vi "broadcast_ping.vi"() -> ()   [LabVIEW 2015]
uses:
  dxl_x86_c.lvlib/dxl_x86_c.lvlib
panel:
  in  "dynamixel_id_list":string[][](table)
  in  "device_name":string="COM8"
  out "protocol_version":dbl=2.0
  out "port_num":i32
  in  "baud_rate":i32=1000000
  # "read_write.vi\n\nCreated on: 2016. 6. 8\nAuthor: Leon Ryu Woon Jung\n\n*********     Read and Write Example      *********\n\n\nAvailable DXL model on this example : All models using Protocol 1.0\nThis example is designed for using a Dynamixel MX-28, and an USB2DYNAMIXEL.\nTo use another Dynamixel model, such as X series, see their details in E-Manual(support.robotis.com) \n   and edit \"numeric control\"s seen left with \"Edit Text\" tool.\nBe sure that Dynamixel MX properties are already set as %% ID : 1 / Baudnum : 1 (Baudrate : 1000000 [1M])\n\n1. Run example by click above \"Run\" button (below \"Edit\" menu).\n2. Drag \"dial\" then you may see the Dynamixel and \"knob\" rotating\n3. To finish the example, press \"terminate\" button."
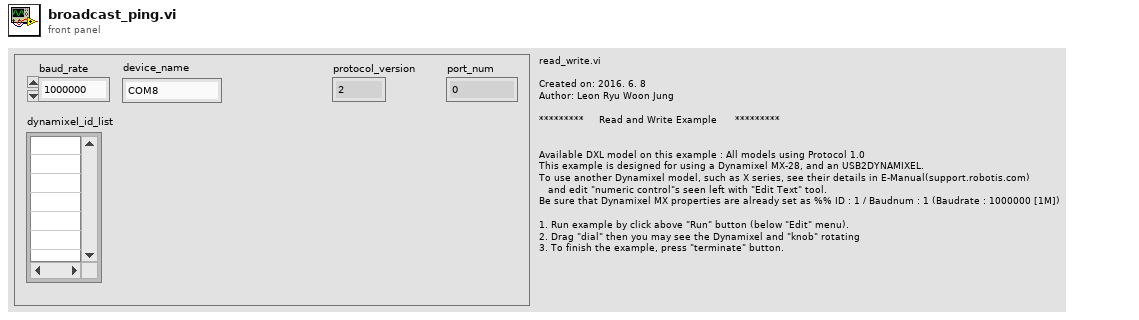
[diagram p1: front panel]
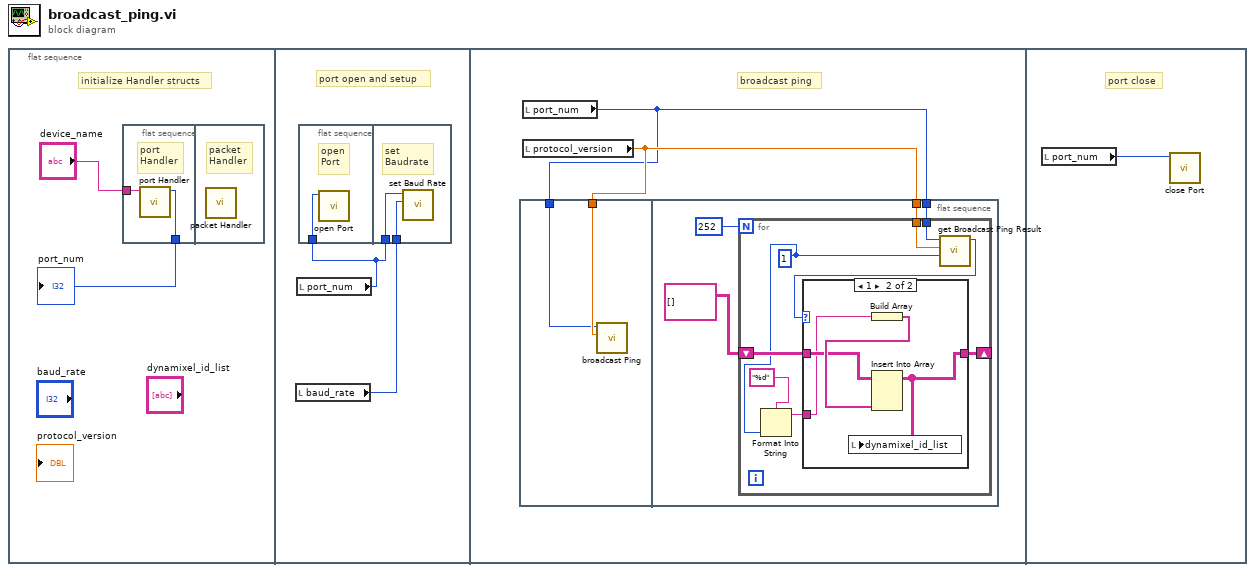
[diagram p0: block diagram]
diagram:
  n1 = flat-sequence {
    frame #0 {
      # "initialize Handler structs"
      n2 = flat-sequence {
        tunnel: [w4] -> w2
        tunnel: "device_name" -> [w3]
        frame #0 {
          # "port\nHandler"
          n3 = call "port Handler.vi"("port_name"=w3) -> ("function return"=w4:i32)  [unwired: 10 in]
        }
        frame #1 {
          # "packet\nHandler"
          n4 = call "packet Handler.vi"() -> ()  [unwired: 12 in]
        }
      }
      "port_num" <- w2
    }
    frame #1 {
      # "port open and setup"
      n5 = local read "baud_rate"() -> (w5:i32)
      n6 = local read "port_num"() -> (w6:i32)
      n7 = flat-sequence {
        tunnel: w6 -> [w7]
        tunnel: w6 -> [w9]
        tunnel: w5 -> [w8]
        frame #0 {
          # "open\nPort"
          n8 = call "open Port.vi"("port_num"=w7) -> ()  [unwired: 10 in, 1 out]
        }
        frame #1 {
          # "set\nBaudrate"
          n9 = call "set Baud Rate.vi"("baudrate"=w8, "port_num"=w9) -> ()  [unwired: 9 in, 1 out]
        }
      }
    }
    frame #2 {
      # "broadcast ping"
      n10 = flat-sequence {
        tunnel: w11 -> [w13]
        tunnel: w10 -> [w12]
        tunnel: w11 -> [w16]
        tunnel: w10 -> [w15]
        frame #0 {
          n11 = call "broadcast Ping.vi"("protocol_version"=w13, "port_num"=w12) -> ()  [unwired: 10 in]
        }
        frame #1 {
          n12 = for {
            N: 252 -> [_]
            tunnel: w16 -> [w24]
            tunnel: w15 -> [w23]
            shift-right: [w21] -> _
            shift-left: string[][] [] -> [w22]
            w18 = 1
            n13 = Format Into String(format string="%d", w18) -> (resulting string=w19:string)  [unwired: 2 in, 1 out]
            n14 = call "get Broadcast Ping Result.vi"("id"=w18, "protocol_version"=w24, "port_num"=w23) -> ("function return"=w25:u8)  [unwired: 8 in]
            n15 = case shown="1" w25 {
              tunnel: w22 -> [w26 w29]
              tunnel: [w26 w27] -> w21
              tunnel: w19 -> [_ w28]
              frame 0, Default {
              }
              frame 1 {
                n16 = Build Array(w28) -> (w30:string[])
                n17 = Insert Into Array(array=w29, new element=w30) -> (w27:string[][])  [unwired: 2 in]
                n18 = local write "dynamixel_id_list"(w27) -> ()
              }
            }
          }
        }
      }
      n19 = local read "port_num"() -> (w10:i32)
      n20 = local read "protocol_version"() -> (w11:dbl)
    }
    frame #3 {
      # "port close"
      n21 = local read "port_num"() -> (w31:i32)
      n22 = call "close Port.vi"("port_num"=w31) -> ()  [unwired: 11 in]
    }
  }
